vi "FileDependency.Create.vi"(8 "error in (no error)":errorcluster, 9 "DLL Path":path, 10 "DLL Property Name":string, 11 "Item Ref in":T1 format="%.0x") -> (0 "error out":errorcluster, 3 "Item Ref out":T1 format="%.0x")   [LabVIEW 2019, in "Protection and Counter Addon System Explorer.lvlib"]
uses:
  Protection and Counter Addon System Explorer.lvlib
  <vilib>/NI VeriStand/Custom Device API/Custom Device Item Ref.ctl
  <vilib>/NI/NI VeriStand Advanced SysDef API/_Types/Property.DependentFile.ctl
  Shared/SubVIs/GUID Lookup.vi
  <vilib>/NI/NI VeriStand Advanced SysDef API/_SubVIs/SysDef.Property.Set.DependentFile.vi
  <vilib>/NI/NI VeriStand Advanced SysDef API/SysDef API/Advanced System Definition.lvlib
  Shared/Protection and Counter Addon Shared.lvlib
  <vilib>/NI VeriStand/Custom Device API/Custom Device API.lvlib
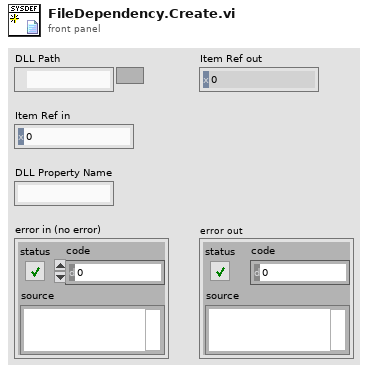
[diagram p1: front panel]
types:
  T1 = typedef "Custom Device API.lvlib/Custom Device Item Ref.ctl" = u64
  T2 = typedef "Advanced System Definition.lvlib/Property.DependentFile.ctl" = cluster{"Original Path":path, "Version":string, "RTDestination":path, "ForceDownload":bool, "SupportedTarget":string, "MD5":string}
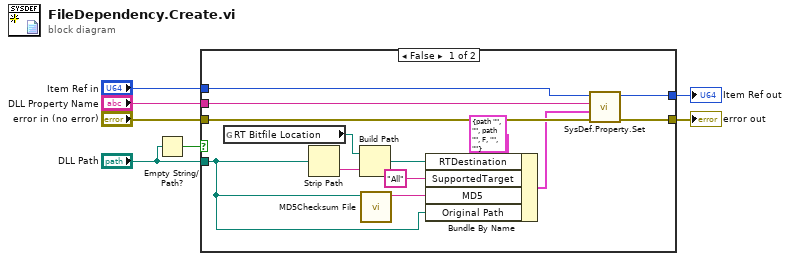
[diagram p0: block diagram]
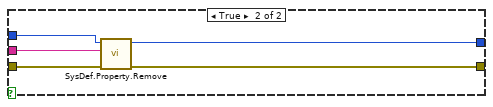
[diagram p2: hidden frame]
diagram:
  n1 = Empty String/Path?(string/path="DLL Path") -> (empty?=w6:bool)
  n2 = case shown="False" w6 {
    tunnel: "error in (no error)" -> [w20 w24]
    tunnel: [w19 w23] -> w3
    tunnel: [w18 w22] -> w4
    tunnel: "Item Ref in" -> [w17 w25]
    tunnel: "DLL Property Name" -> [w16 w21]
    tunnel: "DLL Path" -> [w8 _]
    frame False {
      n3 = global read "GUID Lookup.vi" "RT Bitfile Location"() -> (w15:path)
      n4 = Strip Path(path=w8) -> (name=w14:string)  [unwired: 1 out]
      n5 = Build Path(base path=w15, name or relative path=w14) -> (appended path=w13:path)
      n6 = call <vilib>:"MD5Checksum File.vi"("Path"=w8) -> ("MD5 message-digest"=w11:string)  [unwired: 9 in, 1 out]
      n7 = Bundle By Name(cluster=T2 {"Original Path"=path "", "Version"="", "RTDestination"=path "", "ForceDownload"=FALSE, "SupportedTarget"="", "MD5"=""} ("Value"), "RTDestination"=w13, "SupportedTarget"="All", "MD5"=w11, "Original Path"=w8) -> (w9:T2)
      n8 = call-poly <vilib>:"SysDef.Property.Set.vi"("error in (no error)"=w20, "Value"=w9, "Property Name"=w16, "nodeID"=w17) -> ("error out"=w19:errorcluster, "nodeID out"=w18:u64)  [unwired: 6 in]
    }
    frame True {
      n9 = call <vilib>:"SysDef.Property.Remove.vi"("error in (no error)"=w24, "Property Name"=w21, "nodeID"=w25) -> ("error out"=w23:errorcluster, "nodeID out"=w22:u64)  [unwired: 6 in, 1 out]
    }
  }
  "Item Ref out" <- w4
  "error out" <- w3
